vi "Autonomous Independent.vi"() -> ()   [LabVIEW 2011]
doc: "This VI is called when autonomous begins, and will automatically be terminated when autonomous ends. You can carry out timed or sensor driven robot movement independently without needing to return to the caller."
uses:
  Robot Global Data.vi
panel:
  in  "Speed":dbl=0.75
  in  "Distance":dbl=50.0
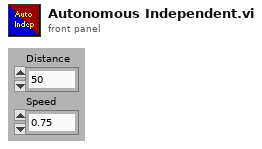
[diagram p1: front panel]
types:
  T1 = cluster{"Autonomous Delay":dbl, "Autonomous Mode":enum16{"Front Of Key", "Middle of Key (SEA)", "Back of Key", "Bridge", "Disable"}}
  T2 = enum16{"Front Of Key", "Middle of Key (SEA)", "Back of Key", "Bridge", "Disable"}
  T3 = cluster{"Left Arm":dbl, "Right Arm":dbl, "Head Right":bool, "Head Left":bool, "Right Leg to Right":bool, "Left Leg to Left":bool, "Right Leg Forward":bool, "Right Leg Back":bool, "Left Leg Forward":bool, "Left Leg Back":bool, "Enable":bool, "Distance":dbl, "Enable Override?":bool, "FIRE!!!!":bool}
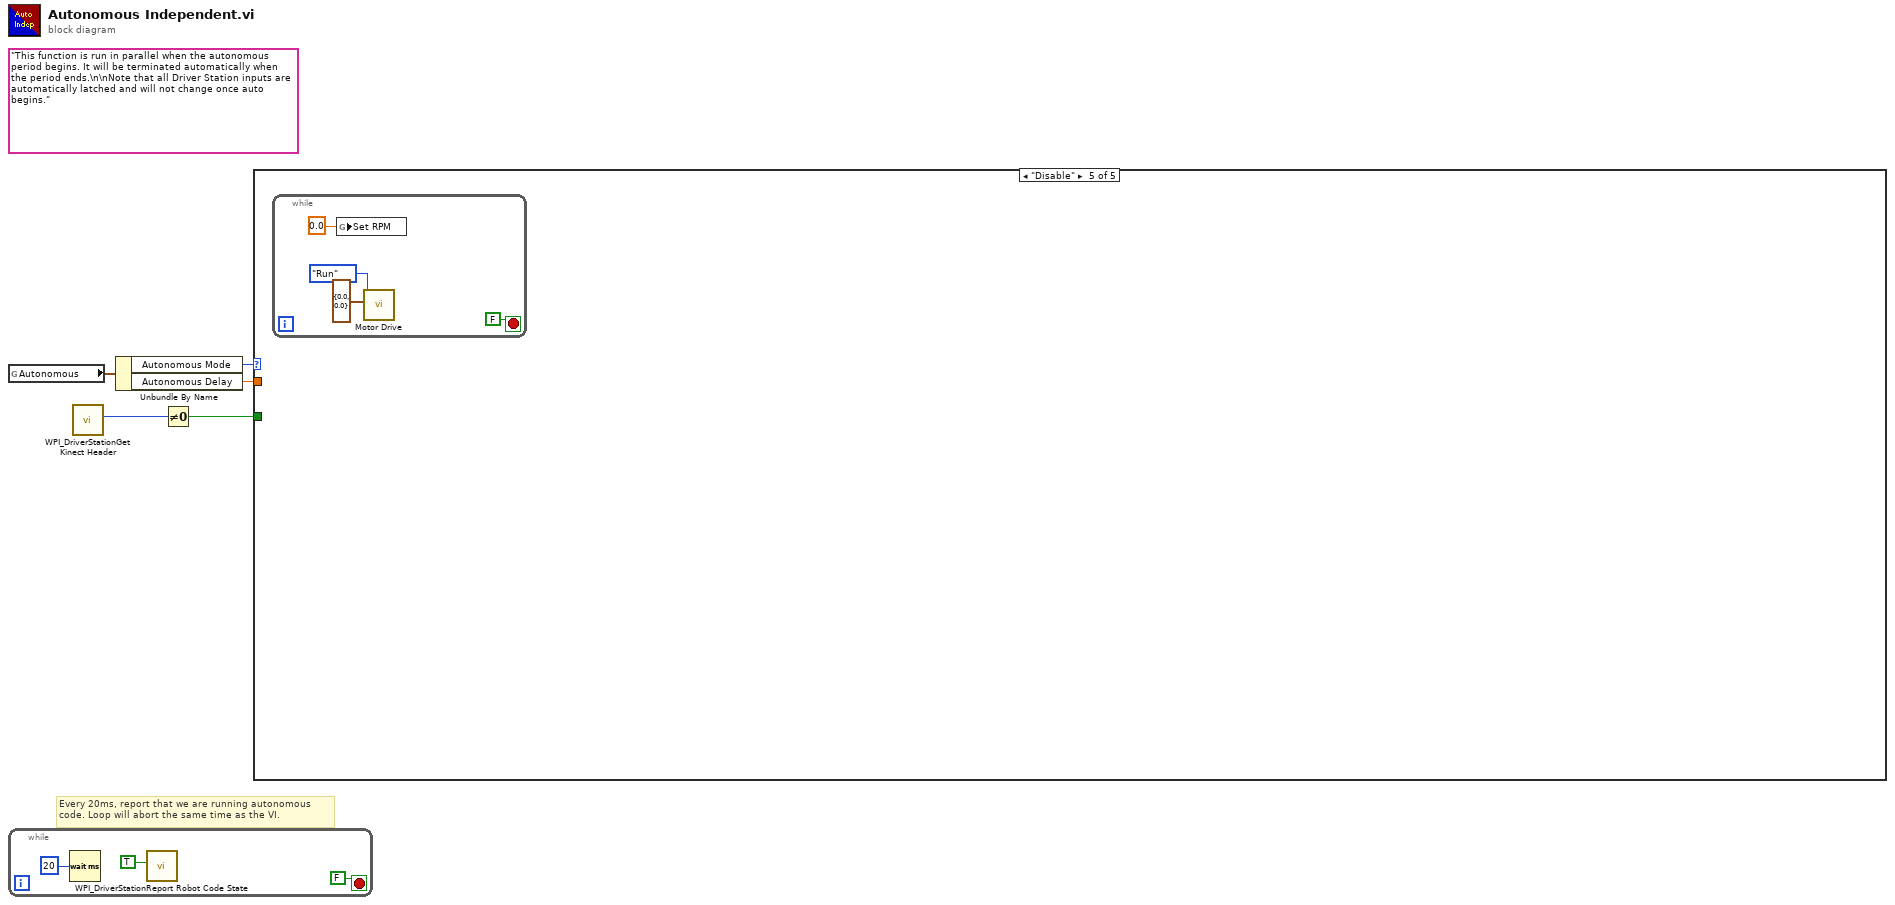
[diagram p0: block diagram]
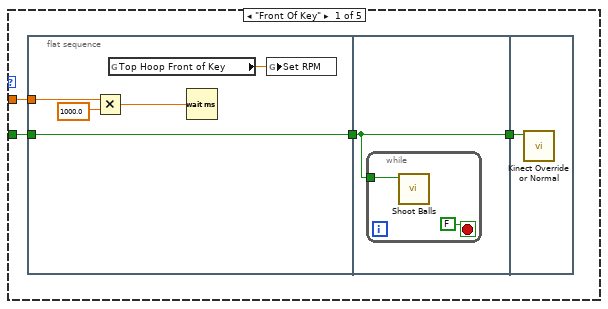
[diagram p2: hidden frame]
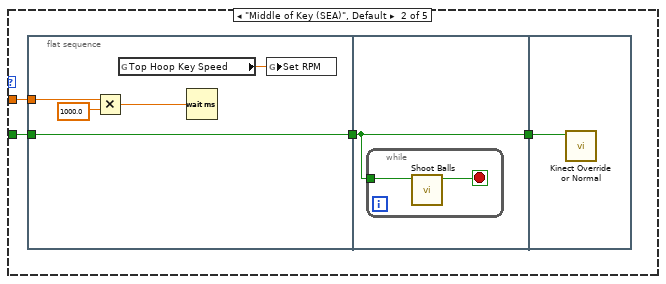
[diagram p3: hidden frame]
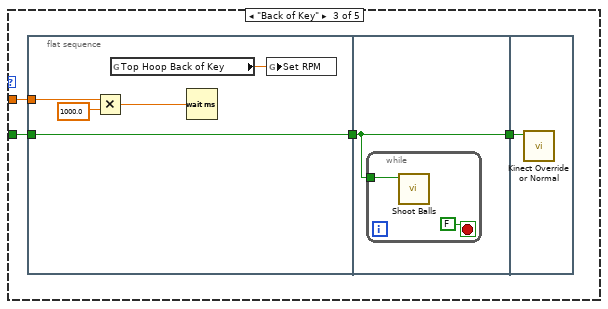
[diagram p4: hidden frame]
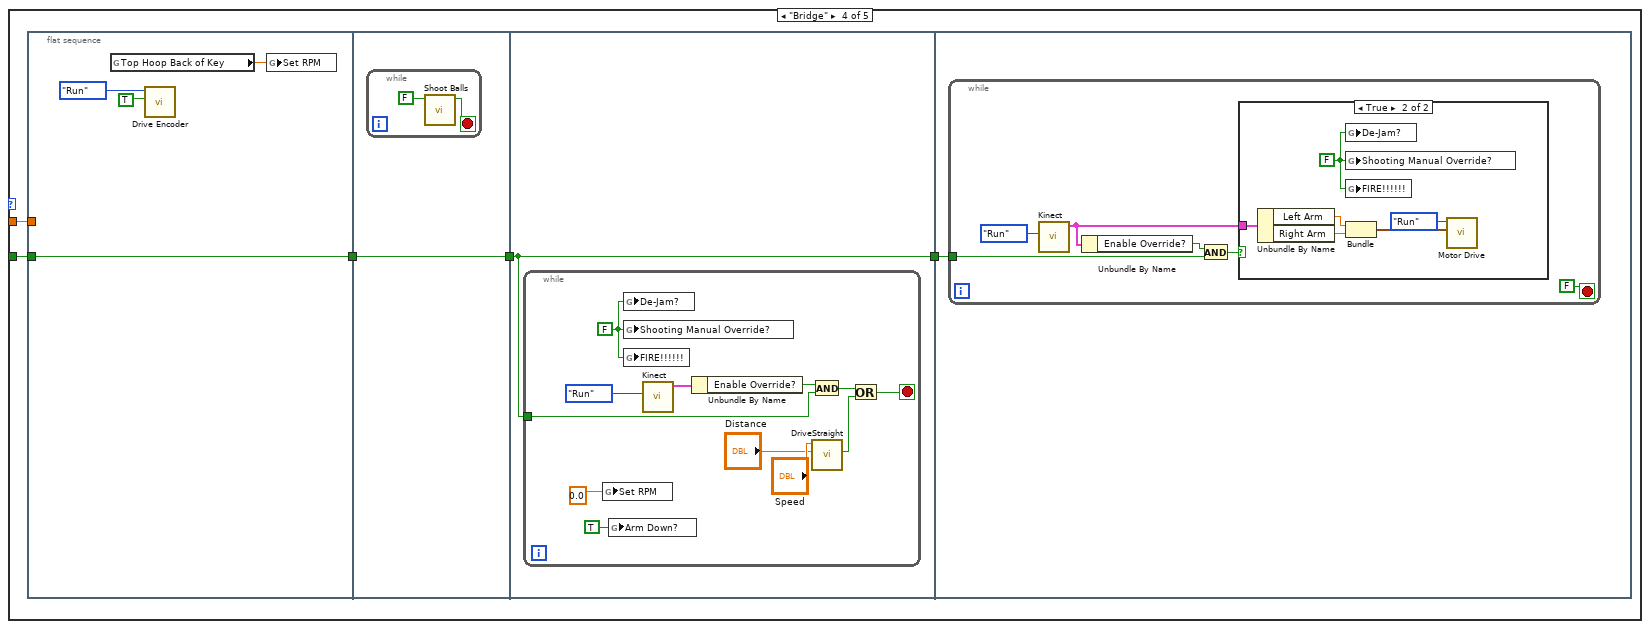
[diagram p5: hidden frame]
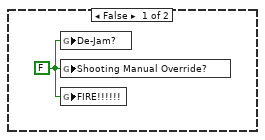
[diagram p6: hidden frame]
diagram:
  (unwired) "This function is run in parallel when the autonomous period begins. It will be terminated automatically when the period ends.\n\nNote that all Driver Station inputs are automatically latched and will not change once auto begins."
  # "Every 20ms, report that we are running autonomous\ncode. Loop will abort the same time as the VI."
  n1 = global read "Robot Global Data.vi" "Autonomous"() -> (w5:T1)
  n2 = while {
    stop <- FALSE stop-if-true
    n3 = Wait (ms)(milliseconds to wait=u32 20) -> ()  [unwired: 1 out]
    n4 = call <vilib>:"WPI_DriverStationReport Robot Code State.vi"("Autonomous"=TRUE) -> ()  [unwired: 10 in, 1 out]
  }
  n5 = call <vilib>:"WPI_DriverStationGet Kinect Header.vi"() -> ("NumPlayers"=w2:i8)  [unwired: 6 in, 5 out]
  n6 = Unbundle By Name(w5) -> ("Autonomous Mode"=w4:T2, "Autonomous Delay"=w3:dbl)
  n7 = Not Equal To 0?(x=w2) -> (x != 0?=w1:bool)
  n8 = case shown="\"Disable\"" w4 {
    tunnel: w3 -> [w12 w25 w38 w52 _]
    tunnel: w1 -> [w11 w23 w36 w50 _]
    frame "Front Of Key" {
      n9 = flat-sequence {
        tunnel: w12 -> [w14]
        tunnel: w11 -> [w13]
        tunnel: [w13] -> w10
        tunnel: w10 -> [w18]
        tunnel: [w18] -> w9
        tunnel: w9 -> [w21]
        frame #0 {
          n10 = Multiply(x=w14, y=1000.0) -> (x*y=w15:dbl)
          n11 = global read "Robot Global Data.vi" "Top Hoop Front of Key"() -> (w17:dbl)
          n12 = Wait (ms)(milliseconds to wait=w15) -> ()  [unwired: 1 out]
          n13 = global write "Robot Global Data.vi" "Set RPM"(w17) -> ()
        }
        frame #1 {
          n14 = while {
            tunnel: w18 -> [w19]
            stop <- FALSE stop-if-true
            n15 = call "Shoot Balls.vi"("Use Kinect?"=w19) -> ()  [unwired: 10 in, 1 out]
          }
        }
        frame #2 {
          n16 = call "Kinect Override or Normal.vi"("KinectEnabled?"=w21) -> ()  [unwired: 11 in]
        }
      }
    }
    frame "Middle of Key (SEA)", Default {
      n17 = flat-sequence {
        tunnel: w25 -> [w27]
        tunnel: [w26] -> w24
        tunnel: w23 -> [w26]
        tunnel: w24 -> [w31]
        tunnel: [w31] -> w22
        tunnel: w22 -> [w34]
        frame #0 {
          n18 = Multiply(x=w27, y=1000.0) -> (x*y=w28:dbl)
          n19 = global read "Robot Global Data.vi" "Top Hoop Key Speed"() -> (w30:dbl)
          n20 = Wait (ms)(milliseconds to wait=w28) -> ()  [unwired: 1 out]
          n21 = global write "Robot Global Data.vi" "Set RPM"(w30) -> ()
        }
        frame #1 {
          n22 = while {
            tunnel: w31 -> [w33]
            stop <- w32 stop-if-true
            n23 = call "Shoot Balls.vi"("Use Kinect?"=w33) -> ("Shot All Balls?"=w32:bool)  [unwired: 10 in]
          }
        }
        frame #2 {
          n24 = call "Kinect Override or Normal.vi"("KinectEnabled?"=w34) -> ()  [unwired: 11 in]
        }
      }
    }
    frame "Back of Key" {
      n25 = flat-sequence {
        tunnel: w38 -> [w40]
        tunnel: w36 -> [w39]
        tunnel: [w39] -> w37
        tunnel: w37 -> [w44]
        tunnel: [w44] -> w35
        tunnel: w35 -> [w47]
        frame #0 {
          n26 = Multiply(x=w40, y=1000.0) -> (x*y=w41:dbl)
          n27 = global read "Robot Global Data.vi" "Top Hoop Back of Key"() -> (w43:dbl)
          n28 = Wait (ms)(milliseconds to wait=w41) -> ()  [unwired: 1 out]
          n29 = global write "Robot Global Data.vi" "Set RPM"(w43) -> ()
        }
        frame #1 {
          n30 = while {
            tunnel: w44 -> [w45]
            stop <- FALSE stop-if-true
            n31 = call "Shoot Balls.vi"("Use Kinect?"=w45) -> ()  [unwired: 10 in, 1 out]
          }
        }
        frame #2 {
          n32 = call "Kinect Override or Normal.vi"("KinectEnabled?"=w47) -> ()  [unwired: 11 in]
        }
      }
    }
    frame "Bridge" {
      n33 = flat-sequence {
        tunnel: w52 -> [_]
        tunnel: [w53] -> w51
        tunnel: w50 -> [w53]
        tunnel: w51 -> [w57]
        tunnel: [w57] -> w48
        tunnel: [w60] -> w49
        tunnel: w48 -> [w60]
        tunnel: w49 -> [w73]
        frame #0 {
          n34 = global read "Robot Global Data.vi" "Top Hoop Back of Key"() -> (w56:dbl)
          n35 = call "Drive Encoder.vi"("Reset"=TRUE, "Enum"=enum16{"Init", "Run", "End"}."Run") -> ()  [unwired: 9 in, 1 out]
          n36 = global write "Robot Global Data.vi" "Set RPM"(w56) -> ()
        }
        frame #1 {
          n37 = while {
            stop <- w59 stop-if-true
            n38 = call "Shoot Balls.vi"("Use Kinect?"=FALSE) -> ("Shot All Balls?"=w59:bool)  [unwired: 10 in]
          }
        }
        frame #2 {
          n39 = while {
            tunnel: w60 -> [w67]
            stop <- w64 stop-if-true
            w63 = FALSE ("De-Jam?")
            n40 = global write "Robot Global Data.vi" "Set RPM"(0.0 ("Set RPM")) -> ()
            n41 = global write "Robot Global Data.vi" "Arm Down?"(TRUE ("Arm Down?")) -> ()
            n42 = global write "Robot Global Data.vi" "De-Jam?"(w63) -> ()
            n43 = global write "Robot Global Data.vi" "Shooting Manual Override?"(w63) -> ()
            n44 = global write "Robot Global Data.vi" "FIRE!!!!!!"(w63) -> ()
            n45 = call "Kinect.vi"("Mode"=enum16{"Init", "Run", "End"}."Run") -> ("Kinect"=w69:T3)  [unwired: 10 in]
            n46 = Unbundle By Name(w69) -> ("Enable Override?"=w68:bool)
            n47 = And(x=w68, y=w67) -> (x .and. y?=w66:bool)
            n48 = call "DriveStraight.vi"("Distance"="Distance", "Speed"="Speed") -> ("At Distance"=w65:bool)  [unwired: 9 in]
            n49 = Or(x=w66, y=w65) -> (x .or. y?=w64:bool)
          }
        }
        frame #3 {
          n50 = while {
            tunnel: w73 -> [w76]
            stop <- FALSE stop-if-true
            n51 = call "Kinect.vi"("Mode"=enum16{"Init", "Run", "End"}."Run") -> ("Kinect"=w74:T3)  [unwired: 10 in]
            n52 = Unbundle By Name(w74) -> ("Enable Override?"=w77:bool)
            n53 = And(x=w77, y=w76) -> (x .and. y?=w75:bool)
            n54 = case shown="True" w75 {
              tunnel: w74 -> [_ w86]
              frame False {
                w80 = FALSE ("De-Jam?")
                n55 = global write "Robot Global Data.vi" "De-Jam?"(w80) -> ()
                n56 = global write "Robot Global Data.vi" "Shooting Manual Override?"(w80) -> ()
                n57 = global write "Robot Global Data.vi" "FIRE!!!!!!"(w80) -> ()
              }
              frame True {
                w82 = FALSE ("De-Jam?")
                n58 = Unbundle By Name(w86) -> ("Left Arm"=w84:dbl, "Right Arm"=w83:dbl)
                n59 = global write "Robot Global Data.vi" "De-Jam?"(w82) -> ()
                n60 = global write "Robot Global Data.vi" "Shooting Manual Override?"(w82) -> ()
                n61 = global write "Robot Global Data.vi" "FIRE!!!!!!"(w82) -> ()
                n62 = Bundle("Left Arm"=w84, "Right Arm"=w83) -> (w85:cluster{"Left Arm":dbl, "Right Arm":dbl})  [unwired: 1 in]
                n63 = call "Motor Drive.vi"("Motor Input"=w85, "Enum"=enum16{"Init", "Run", "SetBrakeCoast", "End"}."Run") -> ()  [unwired: 10 in]
              }
            }
          }
        }
      }
    }
    frame "Disable" {
      n64 = while {
        stop <- FALSE stop-if-true
        n65 = global write "Robot Global Data.vi" "Set RPM"(0.0 ("Set RPM")) -> ()
        n66 = call "Motor Drive.vi"("Motor Input"=cluster{"Left Drive":dbl, "Right Drive":dbl} {"Left Drive"=0.0, "Right Drive"=0.0}, "Enum"=enum16{"Init", "Run", "SetBrakeCoast", "End"}."Run") -> ()  [unwired: 10 in]
      }
    }
  }
